vi "tm450_dcimgrecorder.vi"() -> ()   [LabVIEW 2023, in "HamamatsuCam.lvlib" / "HamamatsuCam.lvclass"]
uses:
  HamamatsuCam/HamamatsuCam/HamamatsuCam.lvclass
panel:
  in  "Seq Buffer":i32=30
  out "Frames Recorded":i32
  in  "DCIMG Path":path
  in  "Frames":i32=100
  out "Error Out":errorcluster
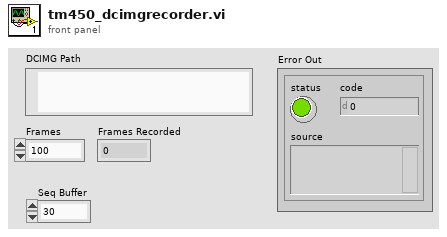
[diagram p1: front panel]
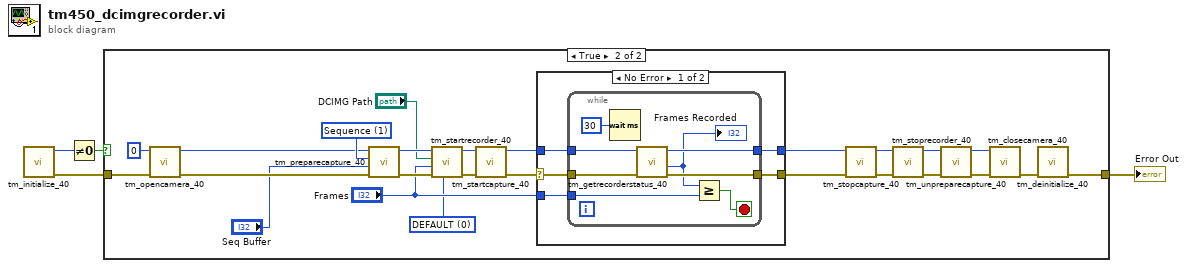
[diagram p0: block diagram]
diagram:
  n1 = call "tm_initialize_40.vi"() -> ("error out"=w1:errorcluster, "Number Of Cameras"=w2:u32)  [unwired: 8 in, 2 out]
  n2 = Not Equal To 0?(x=w2) -> (x != 0?=w4:bool)
  n3 = case shown="True" w4 {
    tunnel: w1 -> [w5 w30]
    tunnel: [w5 w26] -> w3
    frame False {
    }
    frame True {
      w7 = 0 items=["DEFAULT", "NO BUFFERING"] ("Buffering Mode")
      w28 = 1 items=["Snap", "Sequence"] ("Capture mode")
      n4 = call "tm_opencamera_40.vi"("error in (no error)"=w30, "Camera Index"=u32 0) -> ("error out"=w14:errorcluster, "Handle out"=w15:u32)  [unwired: 7 in, 1 out]
      n5 = call "tm_preparecapture_40.vi"("error in (no error)"=w14, "Frames"="Seq Buffer", "Capture mode"=w28, "Handle in"=w15) -> ("error out"=w23:errorcluster, "Handle out"=w22:u32)  [unwired: 4 in, 2 out]
      n6 = call "tm_startrecorder_40.vi"("Buffering Mode"=w7, "error in (no error)"=w23, "frames"="Frames", "File"="DCIMG Path", "Handle in"=w22) -> ("error out"=w21:errorcluster, "Handle out"=w20:u32)  [unwired: 5 in]
      n7 = call "tm_startcapture_40.vi"("error in (no error)"=w21, "Handle in"=w20) -> ("error out"=w19:errorcluster, "Handle out"=w18:u32)  [unwired: 8 in]
      n8 = case shown="No Error" w19 {
        selector: w19 -> [w35 w44]
        tunnel: w18 -> [w34 w45]
        tunnel: [w32 w45] -> w11
        tunnel: [w31 w44] -> w10
        tunnel: "Frames" -> [w33 _]
        frame No Error {
          n9 = while {
            tunnel: w35 -> [w41]
            tunnel: w34 -> [w40]
            tunnel: [w39] -> w31
            tunnel: [w42] -> w32
            tunnel: w33 -> [w43]
            stop <- w36 stop-if-true
            n10 = Wait (ms)(milliseconds to wait=u32 30) -> ()  [unwired: 1 out]
            n11 = call "tm_getrecorderstatus_40.vi"("error in (no error)"=w41, "Handle"=w40) -> ("error out"=w39:errorcluster, "Count"=w38:i32, "Handle"=w42:u32)  [unwired: 6 in, 1 out]
            "Frames Recorded" <- w38
            n12 = Greater Or Equal?(x=w38, y=w43) -> (x >= y?=w36:bool)
          }
        }
        frame Error {
        }
      }
      n13 = call "tm_stopcapture_40.vi"("error in (no error)"=w10, "Handle in"=w11) -> ("error out"=w8:errorcluster, "Handle out"=w9:u32)  [unwired: 8 in]
      n14 = call "tm_stoprecorder_40.vi"("error in (no error)"=w8, "Handle in"=w9) -> ("error out"=w12:errorcluster, "Handle out"=w13:u32)  [unwired: 8 in]
      n15 = call "tm_unpreparecapture_40.vi"("error in (no error)"=w12, "Handle in"=w13) -> ("error out"=w25:errorcluster, "Handle out"=w24:u32)  [unwired: 8 in]
      n16 = call "tm_closecamera_40.vi"("error in (no error)"=w25, "Handle in"=w24) -> ("error out"=w27:errorcluster)  [unwired: 9 in]
      n17 = call "tm_deinitialize_40.vi"("error in (no error)"=w27) -> ("error out"=w26:errorcluster)  [unwired: 10 in]
    }
  }
  "Error Out" <- w3
